vi "DetPort.vi"(8 "error in (no error)":errorcluster caption="错误输入（无错误）", 11 "DET":bool) -> (0 "error out":errorcluster caption="错误输出")   [LabVIEW 2013]
uses:
  SystemCode/SysControl/Slot.ctl
  <vilib>/Utility/error.llb/Error Cluster From Error Code.vi
  GlobalValue.vi
  <vilib>/ErrorRing/Error Ring.xnode
panel:
  out "Port":string[](array[string])
  in  "退出":bool
  # "1.插好连接线\n2.左侧和右侧测试工位放入并连接好T-BOX待测品。\n3.点击下面按钮等待检测通信接口完成。"
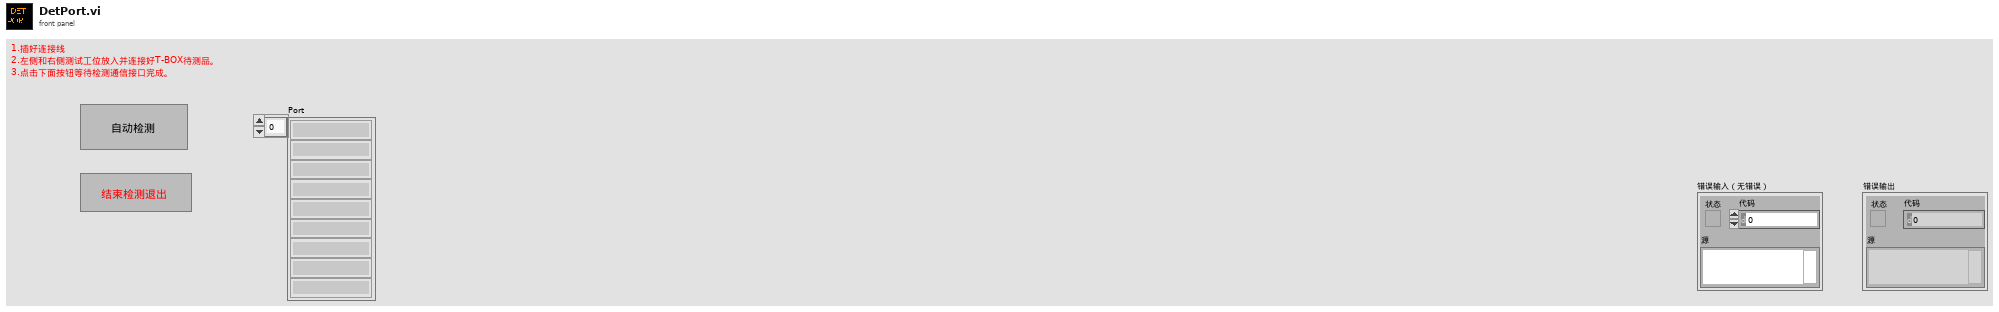
[diagram p1: front panel]
types:
  T1 = typedef "Slot.ctl" = enum16{"Slot1", "Slot2", "Slot3", "Slot4"}
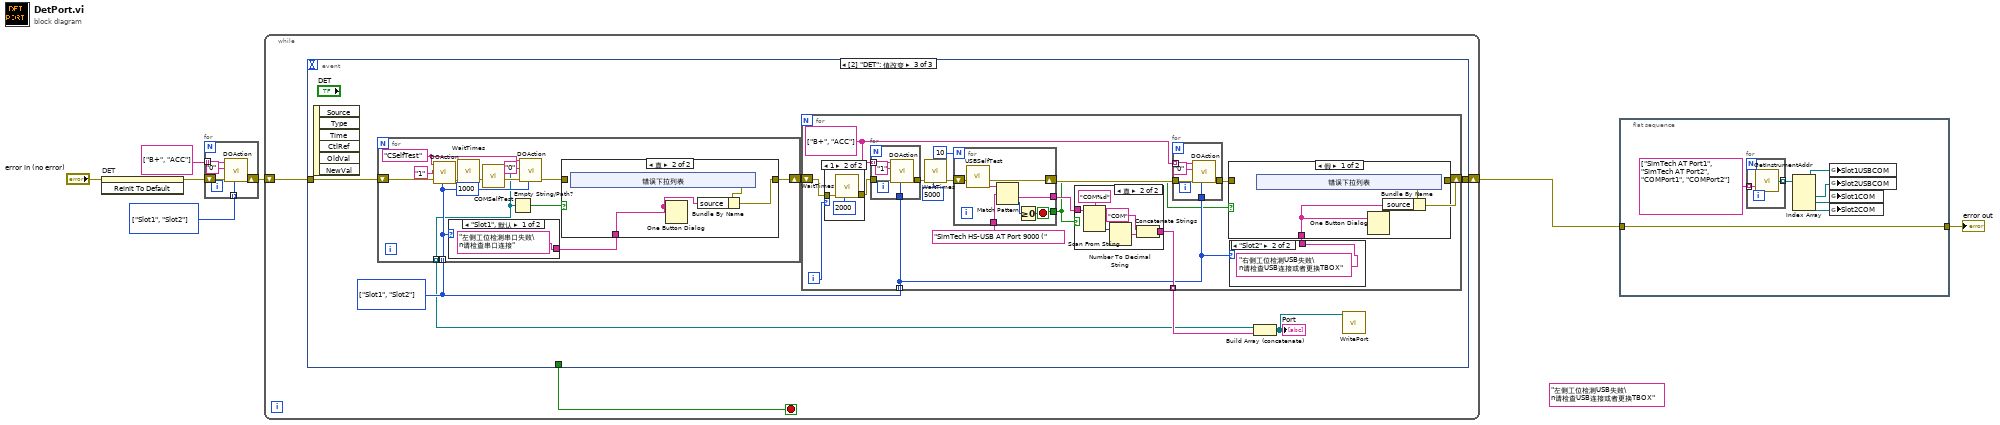
[diagram p0: block diagram]
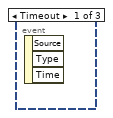
[diagram p2: hidden frame]
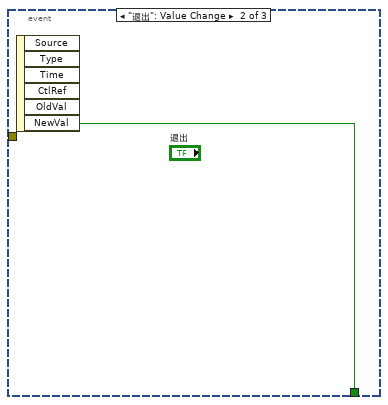
[diagram p3: hidden frame]
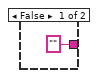
[diagram p5: hidden frame]
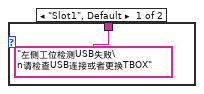
[diagram p6: hidden frame]
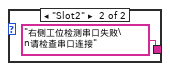
[diagram p8: hidden frame]
diagram:
  w3 = T1[] [enum."Slot1", enum."Slot2"] items=["Slot1", "Slot2", "Slot3", "Slot4"]
  (unwired) "左侧工位检测USB失败\n请检查USB连接或者更换TBOX" ("消息")
  n1 = invoke on="DET" class="Bool" method="Reinit To Default"(error in="error in (no error)") -> (error out=w2:errorcluster)  [unwired: 2 in, 2 out]
  n2 = for {
    tunnel: w3 -> [w12] mode=indexing
    tunnel: string[] ["B+", "ACC"] -> [w11] mode=indexing
    shift-right: [w8] -> w1
    shift-left: w2 -> [w9]
    n3 = call "DOAction.vi"("Slot"=w12, "error in"=w9, "State"="0", "CH"=w11) -> ("error out"=w8:errorcluster)  [unwired: 7 in]
  }
  n4 = while {
    shift-right: [w13] -> w6
    shift-left: w1 -> [w14]
    stop <- w15 stop-if-true
    n5 = event shown="[2] \"DET\": 值改变" {
      selector: _ -> [_ _ _]
      dyn-events: _ -> [_ _ _]
      timeout: _ -> [_ _ _]
      tunnel: [_ w16 _] -> w15
      tunnel: w14 -> [_ _ w23]
      tunnel: [_ _ w21] -> w13
      event Timeout {
        n6 = event-data() -> ()  [unwired: 1 in, 3 out]
      }
      event "退出": Value Change {
        n7 = event-data() -> ("NewVal"=w16:bool)  [unwired: 1 in, 5 out]
      }
      event "DET": Value Change {
        w22 = T1[] [enum."Slot1", enum."Slot2"] items=["Slot1", "Slot2", "Slot3", "Slot4"]
        n8 = event-data() -> ()  [unwired: 1 in, 6 out]
        n9 = for {
          shift-right: [w80] -> w20
          shift-left: w23 -> [w92]
          tunnel: w22 -> [w82] mode=indexing
          tunnel: [w79] -> w18 mode=indexing
          w89 = "CSelfTest" ("CH")
          n10 = call "DOAction.vi"("Slot"=w82, "error in"=w92, "State"="1", "CH"=w89) -> ("error out"=w88:errorcluster)  [unwired: 7 in]
          n11 = case shown="\"Slot1\", 默认" w82 {
            tunnel: ["左侧工位检测串口失败\n请检查串口连接" ("消息") "右侧工位检测串口失败\n请检查串口连接" ("消息")] -> w81
            frame "Slot1", Default {
            }
            frame "Slot2" {
            }
          }
          n12 = call "WaitTimes.vi"("WaitTimes"=u32 1000, "error in (no error)"=w88) -> ("error out"=w87:errorcluster)  [unwired: 9 in]
          n13 = call "COMSelfTest.vi"("error in (no error)"=w87) -> ("error out"=w85:errorcluster, "COMOUT"=w79:refnum<visa-resource-name>)  [unwired: 9 in]
          n14 = Empty String/Path?(string/path=w79) -> (empty?=w83:bool)
          n15 = call "DOAction.vi"("Slot"=w82, "error in"=w85, "State"="0", "CH"=w89) -> ("error out"=w84:errorcluster)  [unwired: 7 in]
          n16 = case shown="真" w83 {
            tunnel: [w95 w97] -> w80
            tunnel: w84 -> [w95 _]
            tunnel: w81 -> [_ w96]
            frame False {
            }
            frame True {
              n17 = xnode "错误下拉列表"() -> ("错误输出"=w98:errorcluster)
              n18 = One Button Dialog(message=w96) -> ()  [unwired: 1 in, 1 out]
              n19 = Bundle By Name(cluster=w98, "source"=w96) -> (w97:errorcluster)
            }
          }
        }
        n20 = for {
          shift-right: [w28] -> w21
          shift-left: w20 -> [w25]
          tunnel: w22 -> [w32] mode=indexing
          tunnel: [w33] -> w19 mode=indexing
          i -> [w26]
          w34 = string[] ["B+", "ACC"]
          n21 = case shown="1" w26 {
            tunnel: w25 -> [w41 w43]
            tunnel: [w41 w42] -> w24
            frame 0, Default {
            }
            frame 1 {
              n22 = call "WaitTimes.vi"("WaitTimes"=u32 2000, "error in (no error)"=w43) -> ("error out"=w42:errorcluster)  [unwired: 9 in]
            }
          }
          n23 = for {
            tunnel: w32 -> [w78]
            tunnel: w34 -> [w77] mode=indexing
            tunnel: w24 -> [w75]
            tunnel: [w74] -> w40
            n24 = call "DOAction.vi"("Slot"=w78, "error in"=w75, "State"="1", "CH"=w77) -> ("error out"=w74:errorcluster)  [unwired: 7 in]
          }
          n25 = call "WaitTimes.vi"("WaitTimes"=u32 5000, "error in (no error)"=w40) -> ("error out"=w27:errorcluster)  [unwired: 9 in]
          n26 = for {
            N: 10 -> [_]
            tunnel: [w71] -> w37
            tunnel: "SimTech HS-USB AT Port 9000 (" ("正则表达式") -> [w70]
            shift-right: [w69] -> w35
            shift-left: w27 -> [w73]
            tunnel: [w68] -> w31
            stop <- w68 stop-if-true
            n27 = call "USBSelfTest.vi"("error in (no error)"=w73) -> ("error out"=w69:errorcluster, "CmdOut"=w67:string)  [unwired: 8 in, 1 out]
            n28 = Match Pattern(string=w67, regular expression=w70) -> (after substring=w71:string, offset past match=w72:i32)  [unwired: 1 in, 2 out]
            n29 = Greater Or Equal To 0?(x=w72) -> (x >= 0?=w68:bool)
          }
          n30 = case shown="真" w31 {
            tunnel: w37 -> [_ w47]
            tunnel: ["" w46] -> w33
            frame False {
            }
            frame True {
              n31 = Scan From String(format string="COM%d" ("格式字符串"), input string=w47) -> (output 1=w50:i32)  [unwired: 3 in, 3 out]
              n32 = Number To Decimal String(number=w50) -> (decimal integer string=w48:string)  [unwired: 1 in]
              n33 = Concatenate Strings("COM" ("字符串"), w48) -> (w46:string)
            }
          }
          n34 = for {
            tunnel: w32 -> [w66]
            tunnel: w34 -> [w65] mode=indexing
            tunnel: w35 -> [w63]
            tunnel: [w62] -> w29
            n35 = call "DOAction.vi"("Slot"=w66, "error in"=w63, "State"="0", "CH"=w65) -> ("error out"=w62:errorcluster)  [unwired: 7 in]
          }
          n36 = case shown="\"Slot2\"" w32 {
            tunnel: ["左侧工位检测USB失败\n请检查USB连接或者更换TBOX" ("消息") "右侧工位检测USB失败\n请检查USB连接或者更换TBOX" ("消息")] -> w30
            frame "Slot1", Default {
            }
            frame "Slot2" {
            }
          }
          n37 = case shown="假" w31 {
            tunnel: [w55 w61] -> w28
            tunnel: w29 -> [_ w61]
            tunnel: w30 -> [w54 _]
            frame False {
              n38 = xnode "错误下拉列表"() -> ("错误输出"=w56:errorcluster)
              n39 = One Button Dialog(message=w54) -> ()  [unwired: 1 in, 1 out]
              n40 = Bundle By Name(cluster=w56, "source"=w54) -> (w55:errorcluster)
            }
            frame True {
            }
          }
        }
        n41 = Build Array (concatenate)(w18, w19) -> (w17:refnum<visa-resource-name>[])
        "Port" <- w17
        n42 = call "WritePort.vi"("Port"=w17) -> ()  [unwired: 10 in, 1 out]
      }
    }
  }
  n43 = flat-sequence {
    tunnel: w6 -> [w103]
    tunnel: [w103] -> w5
    frame #0 {
      n44 = for {
        tunnel: string[] ["SimTech AT Port1", "SimTech AT Port2", "COMPort1", "COMPort2"] -> [w111] mode=indexing
        tunnel: [w110] -> w105 mode=indexing
        n45 = call "GetInstrumentAddr.vi"("String"=w111) -> ("VISA session"=w110:refnum<visa-resource-name>)  [unwired: 1 out]
      }
      n46 = Index Array(array=w105) -> (element #1=w106:refnum<visa-resource-name>, element #2=w107:refnum<visa-resource-name>, element #3=w108:refnum<visa-resource-name>, element #4=w109:refnum<visa-resource-name>)  [unwired: 4 in]
      n47 = global write "GlobalValue.vi" "Slot1USBCOM"(w106) -> ()
      n48 = global write "GlobalValue.vi" "Slot2USBCOM"(w107) -> ()
      n49 = global write "GlobalValue.vi" "Slot1COM"(w108) -> ()
      n50 = global write "GlobalValue.vi" "Slot2COM"(w109) -> ()
    }
  }
  "error out" <- w5
